vi "Att configurações.vi"(0 "Entrada de Configurações":T1={"Simulações"={"Nível Qualidade"="Ótima", "Turno"="Turno 1"}, "Captura de Imagens"={"Pasta com imagens"=path "", "Mostrar imagens capturadas"=FALSE}, "Caminhos"={"Arquivo de log"=path ""}}, 1 "Message Queue":refnum<queue>, 2 "Ler/Gravar":enum16{"Ler", "Gravar"}(ring), 3 "error in (no error)":errorcluster) -> (7 "Saída de configurações":T1={"Simulações"={"Nível Qualidade"="Ótima", "Turno"="Turno 1"}, "Captura de Imagens"={"Pasta com imagens"=path "", "Mostrar imagens capturadas"=FALSE}, "Caminhos"={"Arquivo de log"=path ""}}, 10 "error out":errorcluster)   [LabVIEW 2020, in "Configurações.lvlib"]
doc: "Executa ações definidas para cada configuração que existe no Type Def \"Configurações\".\n\nEsse VI não salva efetivamente as configurações no arquivo .ini ou na memória, ele somente adiciona na fila ações para cada configuração."
uses:
  Message Queue/Message Cluster.ctl
  <vilib>/Utility/config.llb/Read Key (String).vi
  <vilib>/Utility/config.llb/Write Key (String).vi
  Message Queue/Enqueue Message (Single).vi
  <vilib>/Utility/config.llb/Read Key (Boolean).vi
  <vilib>/Utility/config.llb/Read Key (Path).vi
  Message Queue/Message Queue.lvlib
  <vilib>/Utility/config.llb/NI_LVConfig.lvlib
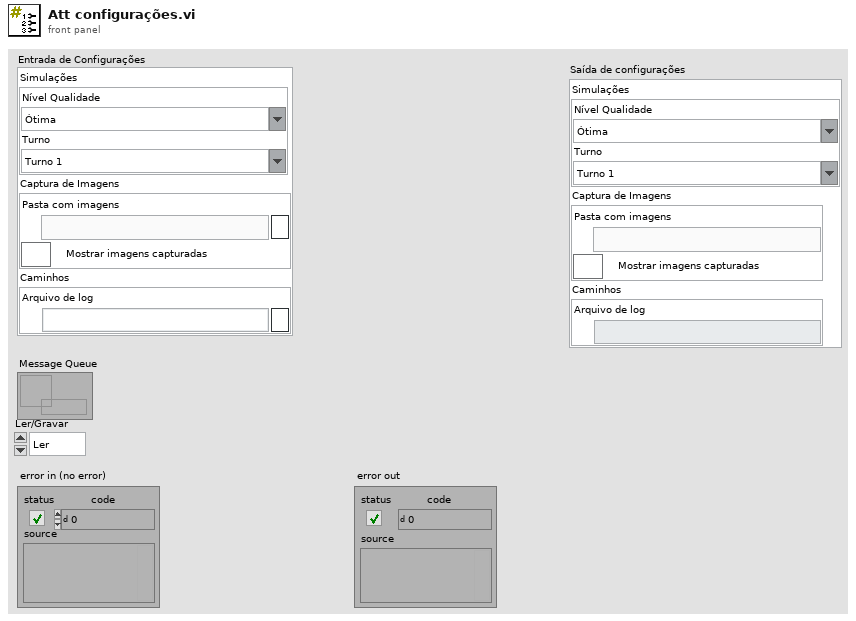
[diagram p1: front panel]
types:
  T1 = typedef "Configurações.lvlib/Configurações padrões.ctl" = cluster{"Simulações":cluster{"Nível Qualidade":string, "Turno":string}, "Captura de Imagens":cluster{"Pasta com imagens":path, "Mostrar imagens capturadas":bool}, "Caminhos":cluster{"Arquivo de log":path}}
  T2 = typedef "NI_LVConfig.lvlib/Config Data RefNum.ctl" = refnum<k1>
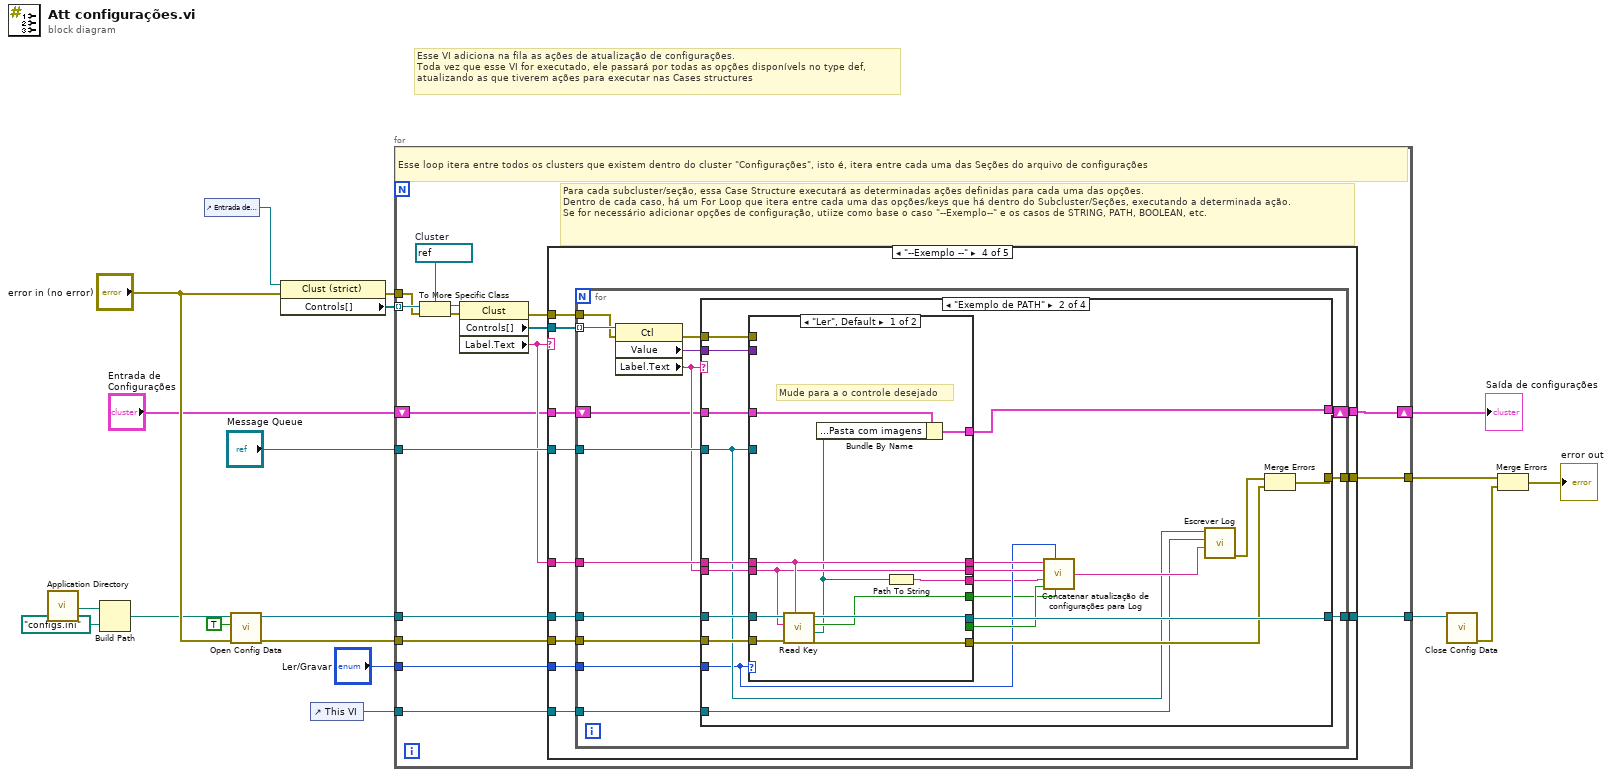
[diagram p0: block diagram]
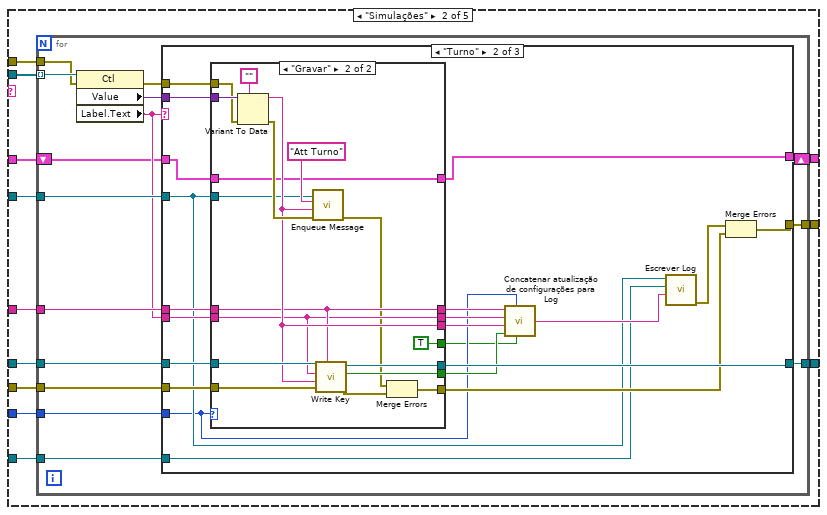
[diagram p3: hidden frame]
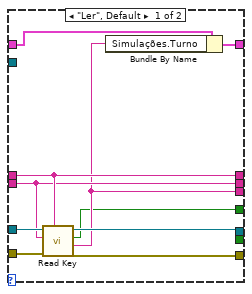
[diagram p5: hidden frame]
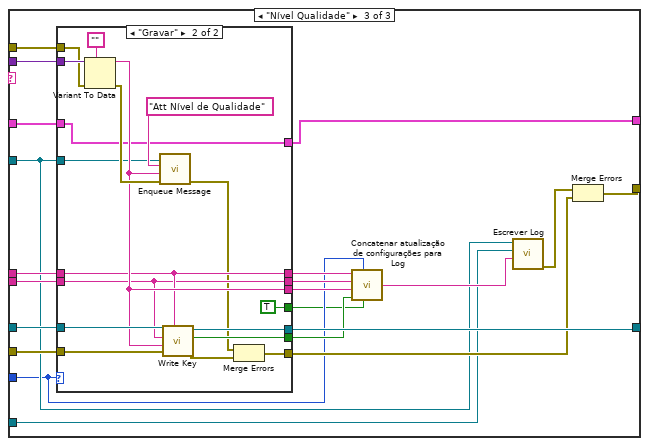
[diagram p6: hidden frame]
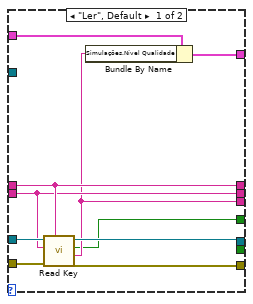
[diagram p7: hidden frame]
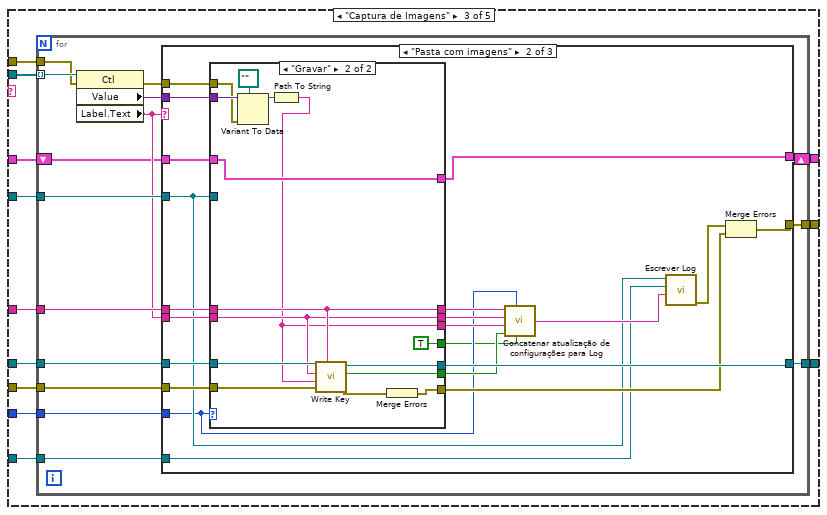
[diagram p8: hidden frame]
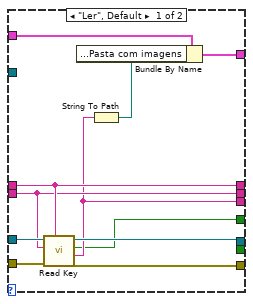
[diagram p10: hidden frame]
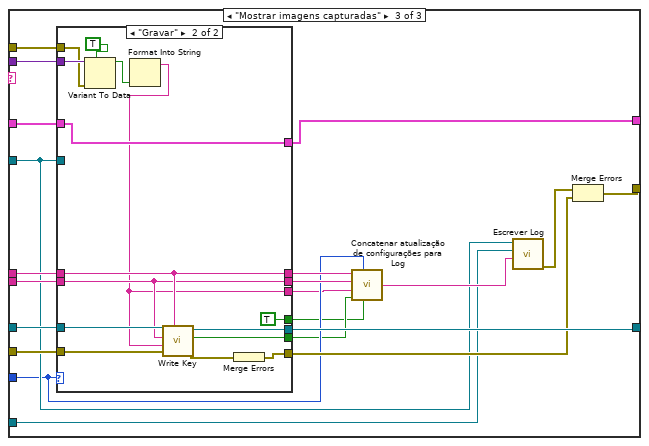
[diagram p11: hidden frame]
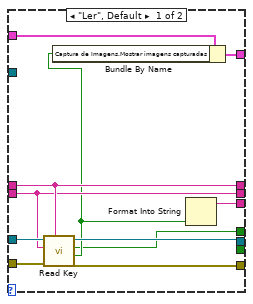
[diagram p12: hidden frame]
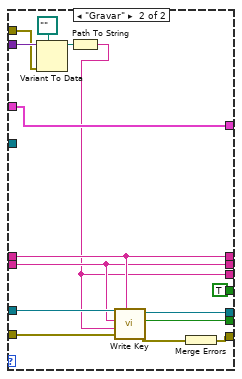
[diagram p14: hidden frame]
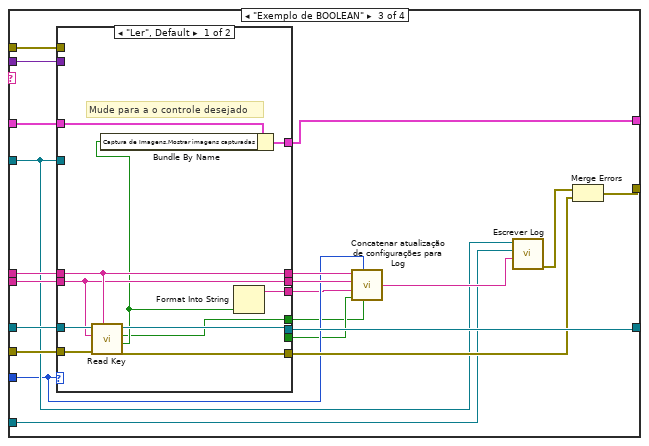
[diagram p15: hidden frame]
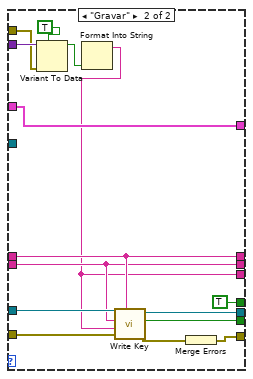
[diagram p16: hidden frame]
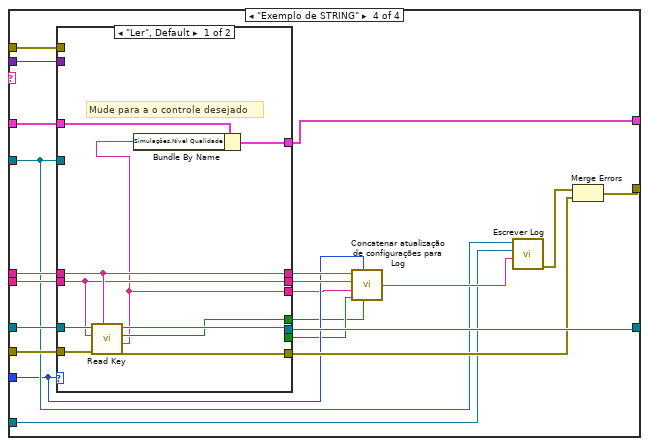
[diagram p17: hidden frame]
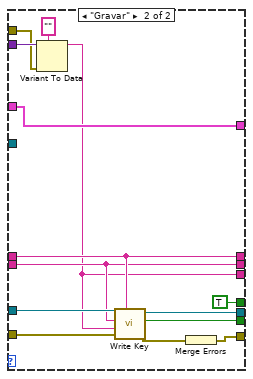
[diagram p18: hidden frame]
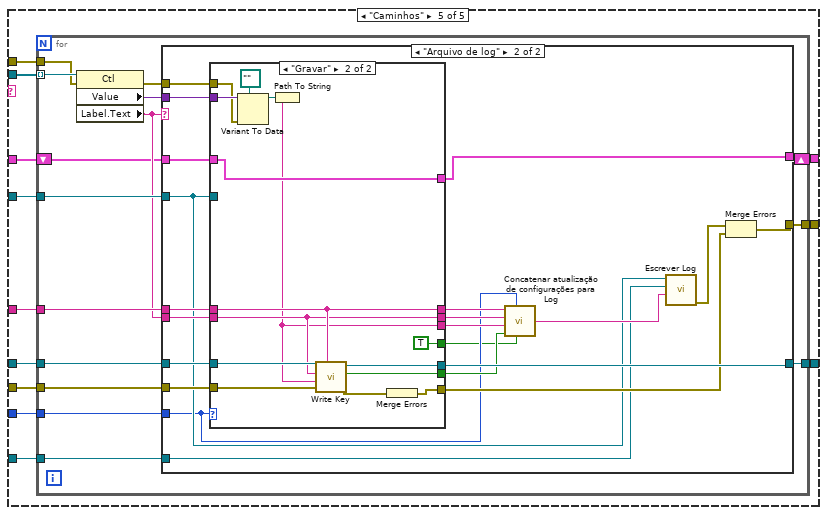
[diagram p19: hidden frame]
diagram:
  # "Esse VI adiciona na fila as ações de atualização de configurações.\nToda vez que esse VI for executado, ele passará por todas as opções disponívels no type def,\natualizando as que tiverem ações para executar nas Cases structures"
  n1 = call <vilib>:"Application Directory.vi"() -> ("Application Directory"=w2:path)
  n2 = Build Path(base path=w2, name or relative path=path "configs.ini") -> (appended path=w1:path)
  n3 = control-ref of="Entrada de Configurações"() -> (w16:refnum<vi>)
  n4 = call <vilib>:"Open Config Data.vi"("error in (no error)"="error in (no error)", "create file if necessary (T)"=TRUE, "configuration file path"=w1) -> ("error out"=w11:errorcluster, "refnum"=w13:T2)  [unwired: 6 in, 1 out]
  n5 = property on="Property Node" class="Clust (strict)"(reference=w16, error in="error in (no error)") -> (error out=w19:errorcluster, "Controls[]"=w18:refnum<vi>[])  [unwired: 1 out]
  n6 = control-ref of="This VI"() -> (w7:refnum<vi>)
  n7 = for {
    tunnel: w18 -> [w36] mode=indexing
    tunnel: w19 -> [w35]
    tunnel: "Message Queue" -> [w29]
    tunnel: [w28] -> w10
    tunnel: w13 -> [w27]
    tunnel: [w26] -> w12
    tunnel: w11 -> [w25]
    tunnel: w7 -> [w23]
    tunnel: "Ler/Gravar" -> [w22]
    shift-right: [w20] -> w4
    shift-left: "Entrada de Configurações" -> [w21]
    w34 = refnum<vi> refnum  # Cluster
    # "Para cada subcluster/seção, essa Case Structure executará as determinadas ações definidas para cada uma das opções.\nDentro de cada caso, há um For Loop que itera entre cada uma das opções/keys que há dentro do Subcluster/Seções, executando a determinada ação.\nSe for necessário adicionar opções de configuração, utiize como base o caso \"--Exemplo--\" e os casos de STRING, PATH, BOOLEAN, etc."
    # "Esse loop itera entre todos os clusters que existem dentro do cluster \"Configurações\", isto é, itera entre cada uma das Seções do arquivo de configurações"
    n8 = To More Specific Class(target class=w34, reference=w36, error in=w35) -> (specific class reference=w33:refnum<vi>, error out=w32:errorcluster)
    n9 = property class="Clust"(reference=w33, error in=w32) -> (error out=w30:errorcluster, "Controls[]"=w31:refnum<vi>[], "Label.Text"=w24:string)  [unwired: 1 out]
    n10 = case shown="\"--Exemplo --\"" w24 {
      tunnel: w31 -> [_ w51 w179 w303 w472]
      tunnel: w30 -> [w39 w50 w178 w302 w471]
      tunnel: w29 -> [_ w49 w177 w301 w470]
      tunnel: [w39 w48 w176 w300 w469] -> w28
      tunnel: w27 -> [w38 w47 w175 w299 w468]
      tunnel: [w38 w46 w174 w298 w467] -> w26
      tunnel: w25 -> [_ w45 w173 w297 w466]
      tunnel: w24 -> [_ w44 w172 w296 w465]
      tunnel: w23 -> [_ w43 w171 w295 w464]
      tunnel: w22 -> [_ w42 w170 w294 w463]
      tunnel: w21 -> [w37 w41 w169 w293 w462]
      tunnel: [w37 w40 w168 w292 w461] -> w20
      frame "Qualquer outra opção", Default {
      }
      frame "Simulações" {
        n11 = for {
          tunnel: w51 -> [w66] mode=indexing
          tunnel: w50 -> [w65]
          tunnel: w49 -> [w64]
          tunnel: [w61] -> w48
          tunnel: w47 -> [w60]
          tunnel: [w59] -> w46
          tunnel: w45 -> [w58]
          tunnel: w44 -> [w57]
          tunnel: w43 -> [w55]
          tunnel: w42 -> [w54]
          shift-right: [w52] -> w40
          shift-left: w41 -> [w53]
          n12 = property class="Ctl"(reference=w66, error in=w65) -> (error out=w62:errorcluster, "Value"=w63:variant, "Label.Text"=w56:string)  [unwired: 1 out]
          n13 = case shown="\"Turno\"" w56 {
            tunnel: w64 -> [_ w75 w124]
            tunnel: w63 -> [_ w90 w139]
            tunnel: w62 -> [w69 w89 w138]
            tunnel: [w69 w80 w129] -> w61
            tunnel: w60 -> [w68 w88 w137]
            tunnel: [w68 w87 w136] -> w59
            tunnel: w58 -> [_ w86 w135]
            tunnel: w57 -> [_ w83 w132]
            tunnel: w56 -> [_ w82 w131]
            tunnel: w55 -> [_ w74 w123]
            tunnel: w54 -> [_ w73 w122]
            tunnel: w53 -> [w67 w72 w121]
            tunnel: [w67 w71 w120] -> w52
            frame "Qualquer outra opção", Default {
            }
            frame "Turno" {
              n14 = case shown="\"Gravar\"" w73 {
                tunnel: w90 -> [_ w118]
                tunnel: w89 -> [_ w116]
                tunnel: w88 -> [w100 w113]
                tunnel: [w99 w112] -> w87
                tunnel: w86 -> [w97 w111]
                tunnel: [_ w110] -> w84
                tunnel: w83 -> [w96 w107]
                tunnel: w82 -> [w95 w106]
                tunnel: [w93 w109] -> w81
                tunnel: [w98 w104] -> w78
                tunnel: w75 -> [_ w108]
                tunnel: [w96 w107] -> w77
                tunnel: [w95 w106] -> w76
                tunnel: [w94 w102] -> w71
                tunnel: w72 -> [w92 w102]
                tunnel: [w91 TRUE ("found?")] -> w70
                frame "Ler", Default {
                  n15 = call-poly <vilib>:"Read Key.vi"("section"=w96, "error in (no error)"=w97, "key"=w95, "refnum"=w100) -> ("error out"=w98:errorcluster, "value"=w93:string, "found?"=w91:bool, "refnum out"=w99:T2)  [unwired: 4 in]
                  n16 = Bundle By Name(cluster=w92, "Simulações.Turno"=w93) -> (w94:T1)
                }
                frame "Gravar" {
                  n17 = Variant To Data(error in=w116, type="", Variant=w118) -> (data=w109:string, error out=w115:errorcluster)
                  n18 = call-poly "Enqueue Message.vi"("error in (no error)"=w115, "Message Data"=w109, "Message"="Att Turno", "Message Queue"=w108) -> ("error out"=w103:errorcluster)  [unwired: 6 in, 1 out]
                  n19 = call-poly <vilib>:"Write Key.vi"("section"=w107, "error in (no error)"=w111, "value"=w109, "key"=w106, "refnum"=w113) -> ("error out"=w105:errorcluster, "found?"=w110:bool, "refnum out"=w112:T2)  [unwired: 4 in]
                  n20 = Merge Errors(w103, w105) -> (w104:errorcluster)
                }
              }
              n21 = call "Concatenar atualização de configurações para Log.vi"("Seção/Key encontrada"=w70, "Leitura/Escrita"=w73, "Key ja existia?"=w84, "Valor"=w81, "Nome da Chave"=w76, "Nome da Seção"=w77) -> ("Texto Concatenado"=w85:string)
              n22 = call "Escrever Log.vi"("Dados para Log"=w85, "VI"=w74, "Queue in"=w75) -> ("error out"=w79:errorcluster)  [unwired: 7 in, 1 out]
              n23 = Merge Errors(w79, w78) -> (w80:errorcluster)
            }
            frame "Nível Qualidade" {
              n24 = case shown="\"Gravar\"" w122 {
                tunnel: w139 -> [_ w167]
                tunnel: w138 -> [_ w165]
                tunnel: w137 -> [w149 w162]
                tunnel: [w148 w161] -> w136
                tunnel: w135 -> [w146 w160]
                tunnel: [_ w159] -> w133
                tunnel: w132 -> [w145 w156]
                tunnel: w131 -> [w144 w155]
                tunnel: [w142 w158] -> w130
                tunnel: [w147 w153] -> w127
                tunnel: w124 -> [_ w157]
                tunnel: [w145 w156] -> w126
                tunnel: [w144 w155] -> w125
                tunnel: [w143 w151] -> w120
                tunnel: w121 -> [w141 w151]
                tunnel: [w140 TRUE ("found?")] -> w119
                frame "Ler", Default {
                  n25 = call-poly <vilib>:"Read Key.vi"("section"=w145, "error in (no error)"=w146, "key"=w144, "refnum"=w149) -> ("error out"=w147:errorcluster, "value"=w142:string, "found?"=w140:bool, "refnum out"=w148:T2)  [unwired: 4 in]
                  n26 = Bundle By Name(cluster=w141, "Simulações.Nível Qualidade"=w142) -> (w143:T1)
                }
                frame "Gravar" {
                  n27 = Variant To Data(error in=w165, type="", Variant=w167) -> (data=w158:string, error out=w164:errorcluster)
                  n28 = call-poly "Enqueue Message.vi"("error in (no error)"=w164, "Message Data"=w158, "Message"="Att Nível de Qualidade", "Message Queue"=w157) -> ("error out"=w152:errorcluster)  [unwired: 6 in, 1 out]
                  n29 = call-poly <vilib>:"Write Key.vi"("section"=w156, "error in (no error)"=w160, "value"=w158, "key"=w155, "refnum"=w162) -> ("error out"=w154:errorcluster, "found?"=w159:bool, "refnum out"=w161:T2)  [unwired: 4 in]
                  n30 = Merge Errors(w152, w154) -> (w153:errorcluster)
                }
              }
              n31 = call "Concatenar atualização de configurações para Log.vi"("Seção/Key encontrada"=w119, "Leitura/Escrita"=w122, "Key ja existia?"=w133, "Valor"=w130, "Nome da Chave"=w125, "Nome da Seção"=w126) -> ("Texto Concatenado"=w134:string)
              n32 = call "Escrever Log.vi"("Dados para Log"=w134, "VI"=w123, "Queue in"=w124) -> ("error out"=w128:errorcluster)  [unwired: 7 in, 1 out]
              n33 = Merge Errors(w128, w127) -> (w129:errorcluster)
            }
          }
        }
      }
      frame "Captura de Imagens" {
        n34 = for {
          tunnel: w179 -> [w194] mode=indexing
          tunnel: w178 -> [w193]
          tunnel: w177 -> [w192]
          tunnel: [w189] -> w176
          tunnel: w175 -> [w188]
          tunnel: [w187] -> w174
          tunnel: w173 -> [w186]
          tunnel: w172 -> [w185]
          tunnel: w171 -> [w183]
          tunnel: w170 -> [w182]
          shift-right: [w180] -> w168
          shift-left: w169 -> [w181]
          n35 = property class="Ctl"(reference=w194, error in=w193) -> (error out=w190:errorcluster, "Value"=w191:variant, "Label.Text"=w184:string)  [unwired: 1 out]
          n36 = case shown="\"Pasta com imagens\"" w184 {
            tunnel: w192 -> [_ w203 w252]
            tunnel: w191 -> [_ w218 w265]
            tunnel: w190 -> [w197 w217 w264]
            tunnel: [w197 w208 w257] -> w189
            tunnel: w188 -> [w196 w216 w263]
            tunnel: [w196 w215 w262] -> w187
            tunnel: w186 -> [_ w214 w261]
            tunnel: w185 -> [_ w211 w259]
            tunnel: w184 -> [_ w210 w258]
            tunnel: w183 -> [_ w202 w251]
            tunnel: w182 -> [_ w201 w250]
            tunnel: w181 -> [w195 w200 w249]
            tunnel: [w195 w199 w248] -> w180
            frame "Qualquer outra opção", Default {
            }
            frame "Pasta com imagens" {
              n37 = case shown="\"Gravar\"" w201 {
                tunnel: w218 -> [_ w244]
                tunnel: w217 -> [_ w243]
                tunnel: w216 -> [w229 w242]
                tunnel: [w228 w241] -> w215
                tunnel: w214 -> [w226 w240]
                tunnel: [_ w239] -> w212
                tunnel: w211 -> [w225 w238]
                tunnel: w210 -> [w224 w237]
                tunnel: [w220 w230] -> w209
                tunnel: [w227 w235] -> w206
                tunnel: w203 -> [_ _]
                tunnel: [w225 w238] -> w205
                tunnel: [w224 w237] -> w204
                tunnel: [w223 w234] -> w199
                tunnel: w200 -> [w222 w234]
                tunnel: [w219 TRUE ("found?")] -> w198
                frame "Ler", Default {
                  n38 = call-poly <vilib>:"Read Key.vi"("section"=w225, "error in (no error)"=w226, "key"=w224, "refnum"=w229) -> ("error out"=w227:errorcluster, "value"=w220:string, "found?"=w219:bool, "refnum out"=w228:T2)  [unwired: 4 in]
                  n39 = String To Path(string=w220) -> (path=w221:path)
                  n40 = Bundle By Name(cluster=w222, "Captura de Imagens.Pasta com imagens"=w221) -> (w223:T1)
                }
                frame "Gravar" {
                  n41 = Variant To Data(error in=w243, type=path "", Variant=w244) -> (data=w231:path)  [unwired: 1 out]
                  n42 = Path To String(path=w231) -> (string=w230:string)
                  n43 = call-poly <vilib>:"Write Key.vi"("section"=w238, "error in (no error)"=w240, "value"=w230, "key"=w237, "refnum"=w242) -> ("error out"=w236:errorcluster, "found?"=w239:bool, "refnum out"=w241:T2)  [unwired: 4 in]
                  n44 = Merge Errors(w236) -> (w235:errorcluster)
                }
              }
              n45 = call "Concatenar atualização de configurações para Log.vi"("Seção/Key encontrada"=w198, "Leitura/Escrita"=w201, "Key ja existia?"=w212, "Valor"=w209, "Nome da Chave"=w204, "Nome da Seção"=w205) -> ("Texto Concatenado"=w213:string)
              n46 = call "Escrever Log.vi"("Dados para Log"=w213, "VI"=w202, "Queue in"=w203) -> ("error out"=w207:errorcluster)  [unwired: 7 in, 1 out]
              n47 = Merge Errors(w207, w206) -> (w208:errorcluster)
            }
            frame "Mostrar imagens capturadas" {
              n48 = case shown="\"Gravar\"" w250 {
                tunnel: w265 -> [_ w291]
                tunnel: w264 -> [_ w290]
                tunnel: w263 -> [w276 w289]
                tunnel: [w275 w288] -> w262
                tunnel: w261 -> [w273 w287]
                tunnel: [_ w286] -> w247
                tunnel: w259 -> [w272 w285]
                tunnel: w258 -> [w271 w284]
                tunnel: [w274 w282] -> w255
                tunnel: w252 -> [_ _]
                tunnel: [w272 w285] -> w254
                tunnel: [w271 w284] -> w253
                tunnel: [w270 w281] -> w248
                tunnel: w249 -> [w268 w281]
                tunnel: [w267 w277] -> w246
                tunnel: [w266 TRUE ("found?")] -> w245
                frame "Ler", Default {
                  n49 = call-poly <vilib>:"Read Key.vi"("section"=w272, "error in (no error)"=w273, "key"=w271, "refnum"=w276) -> ("error out"=w274:errorcluster, "value"=w269:bool, "found?"=w266:bool, "refnum out"=w275:T2)  [unwired: 4 in]
                  n50 = Bundle By Name(cluster=w268, "Captura de Imagens.Mostrar imagens capturadas"=w269) -> (w270:T1)
                  n51 = Format Into String(w269) -> (resulting string=w267:string)  [unwired: 3 in, 1 out]
                }
                frame "Gravar" {
                  n52 = Variant To Data(error in=w290, type=TRUE, Variant=w291) -> (data=w278:bool)  [unwired: 1 out]
                  n53 = Format Into String(w278) -> (resulting string=w277:string)  [unwired: 3 in, 1 out]
                  n54 = call-poly <vilib>:"Write Key.vi"("section"=w285, "error in (no error)"=w287, "value"=w277, "key"=w284, "refnum"=w289) -> ("error out"=w283:errorcluster, "found?"=w286:bool, "refnum out"=w288:T2)  [unwired: 4 in]
                  n55 = Merge Errors(w283) -> (w282:errorcluster)
                }
              }
              n56 = call "Concatenar atualização de configurações para Log.vi"("Seção/Key encontrada"=w245, "Leitura/Escrita"=w250, "Key ja existia?"=w247, "Valor"=w246, "Nome da Chave"=w253, "Nome da Seção"=w254) -> ("Texto Concatenado"=w260:string)
              n57 = call "Escrever Log.vi"("Dados para Log"=w260, "VI"=w251, "Queue in"=w252) -> ("error out"=w256:errorcluster)  [unwired: 7 in, 1 out]
              n58 = Merge Errors(w256, w255) -> (w257:errorcluster)
            }
          }
        }
      }
      frame "--Exemplo --" {
        n59 = for {
          tunnel: w303 -> [w318] mode=indexing
          tunnel: w302 -> [w317]
          tunnel: w301 -> [w316]
          tunnel: [w313] -> w300
          tunnel: w299 -> [w312]
          tunnel: [w311] -> w298
          tunnel: w297 -> [w310]
          tunnel: w296 -> [w309]
          tunnel: w295 -> [w307]
          tunnel: w294 -> [w306]
          shift-right: [w304] -> w292
          shift-left: w293 -> [w305]
          n60 = property class="Ctl"(reference=w318, error in=w317) -> (error out=w314:errorcluster, "Value"=w315:variant, "Label.Text"=w308:string)  [unwired: 1 out]
          n61 = case shown="\"Exemplo de PATH\"" w308 {
            tunnel: w316 -> [_ w328 w376 w423]
            tunnel: w315 -> [_ w342 w389 w436]
            tunnel: w314 -> [w321 w341 w388 w435]
            tunnel: [w321 w333 w381 w428] -> w313
            tunnel: w312 -> [w320 w340 w387 w434]
            tunnel: [w320 w339 w386 w433] -> w311
            tunnel: w310 -> [_ w338 w385 w432]
            tunnel: w309 -> [_ w335 w383 w430]
            tunnel: w308 -> [_ w334 w382 w429]
            tunnel: w307 -> [_ w327 w375 w422]
            tunnel: w306 -> [_ w326 w374 w421]
            tunnel: w305 -> [w319 w325 w373 w420]
            tunnel: [w319 w324 w372 w419] -> w304
            frame "Qualquer outra opção", Default {
            }
            frame "Exemplo de PATH" {
              n62 = case shown="\"Ler\", Default" w326 {
                tunnel: w342 -> [_ w368]
                tunnel: w341 -> [_ w367]
                tunnel: w340 -> [w353 w366]
                tunnel: [w352 w365] -> w339
                tunnel: w338 -> [w350 w364]
                tunnel: [_ w363] -> w336
                tunnel: w335 -> [w349 w362]
                tunnel: w334 -> [w348 w361]
                tunnel: [w351 w359] -> w331
                tunnel: w328 -> [_ _]
                tunnel: [w349 w362] -> w330
                tunnel: [w348 w361] -> w329
                tunnel: [w347 w358] -> w324
                tunnel: w325 -> [w346 w358]
                tunnel: [w345 TRUE ("found?")] -> w323
                tunnel: [w343 w354] -> w322
                frame "Ler", Default {
                  # "Mude para a o controle desejado"
                  n63 = call-poly <vilib>:"Read Key.vi"("section"=w349, "error in (no error)"=w350, "key"=w348, "refnum"=w353) -> ("error out"=w351:errorcluster, "value"=w344:path, "found?"=w345:bool, "refnum out"=w352:T2)  [unwired: 4 in]
                  n64 = Bundle By Name(cluster=w346, "Captura de Imagens.Pasta com imagens"=w344) -> (w347:T1)
                  n65 = Path To String(path=w344) -> (string=w343:string)
                }
                frame "Gravar" {
                  n66 = Variant To Data(error in=w367, type=path "", Variant=w368) -> (data=w355:path)  [unwired: 1 out]
                  n67 = Path To String(path=w355) -> (string=w354:string)
                  n68 = call-poly <vilib>:"Write Key.vi"("section"=w362, "error in (no error)"=w364, "value"=w354, "key"=w361, "refnum"=w366) -> ("error out"=w360:errorcluster, "found?"=w363:bool, "refnum out"=w365:T2)  [unwired: 4 in]
                  n69 = Merge Errors(w360) -> (w359:errorcluster)
                }
              }
              n70 = call "Concatenar atualização de configurações para Log.vi"("Seção/Key encontrada"=w323, "Leitura/Escrita"=w326, "Key ja existia?"=w336, "Valor"=w322, "Nome da Chave"=w329, "Nome da Seção"=w330) -> ("Texto Concatenado"=w337:string)
              n71 = call "Escrever Log.vi"("Dados para Log"=w337, "VI"=w327, "Queue in"=w328) -> ("error out"=w332:errorcluster)  [unwired: 7 in, 1 out]
              n72 = Merge Errors(w332, w331) -> (w333:errorcluster)
            }
            frame "Exemplo de BOOLEAN" {
              n73 = case shown="\"Ler\", Default" w374 {
                tunnel: w389 -> [_ w415]
                tunnel: w388 -> [_ w414]
                tunnel: w387 -> [w400 w413]
                tunnel: [w399 w412] -> w386
                tunnel: w385 -> [w397 w411]
                tunnel: [_ w410] -> w371
                tunnel: w383 -> [w396 w409]
                tunnel: w382 -> [w395 w408]
                tunnel: [w398 w406] -> w379
                tunnel: w376 -> [_ _]
                tunnel: [w396 w409] -> w378
                tunnel: [w395 w408] -> w377
                tunnel: [w394 w405] -> w372
                tunnel: w373 -> [w392 w405]
                tunnel: [w391 w401] -> w370
                tunnel: [w390 TRUE ("found?")] -> w369
                frame "Ler", Default {
                  # "Mude para a o controle desejado"
                  n74 = call-poly <vilib>:"Read Key.vi"("section"=w396, "error in (no error)"=w397, "key"=w395, "refnum"=w400) -> ("error out"=w398:errorcluster, "value"=w393:bool, "found?"=w390:bool, "refnum out"=w399:T2)  [unwired: 4 in]
                  n75 = Bundle By Name(cluster=w392, "Captura de Imagens.Mostrar imagens capturadas"=w393) -> (w394:T1)
                  n76 = Format Into String(w393) -> (resulting string=w391:string)  [unwired: 3 in, 1 out]
                }
                frame "Gravar" {
                  n77 = Variant To Data(error in=w414, type=TRUE, Variant=w415) -> (data=w402:bool)  [unwired: 1 out]
                  n78 = Format Into String(w402) -> (resulting string=w401:string)  [unwired: 3 in, 1 out]
                  n79 = call-poly <vilib>:"Write Key.vi"("section"=w409, "error in (no error)"=w411, "value"=w401, "key"=w408, "refnum"=w413) -> ("error out"=w407:errorcluster, "found?"=w410:bool, "refnum out"=w412:T2)  [unwired: 4 in]
                  n80 = Merge Errors(w407) -> (w406:errorcluster)
                }
              }
              n81 = call "Concatenar atualização de configurações para Log.vi"("Seção/Key encontrada"=w369, "Leitura/Escrita"=w374, "Key ja existia?"=w371, "Valor"=w370, "Nome da Chave"=w377, "Nome da Seção"=w378) -> ("Texto Concatenado"=w384:string)
              n82 = call "Escrever Log.vi"("Dados para Log"=w384, "VI"=w375, "Queue in"=w376) -> ("error out"=w380:errorcluster)  [unwired: 7 in, 1 out]
              n83 = Merge Errors(w380, w379) -> (w381:errorcluster)
            }
            frame "Exemplo de STRING" {
              n84 = case shown="\"Ler\", Default" w421 {
                tunnel: w436 -> [_ w460]
                tunnel: w435 -> [_ w459]
                tunnel: w434 -> [w446 w458]
                tunnel: [w445 w457] -> w433
                tunnel: w432 -> [w443 w456]
                tunnel: [_ w455] -> w418
                tunnel: w430 -> [w442 w454]
                tunnel: w429 -> [w441 w453]
                tunnel: [w444 w451] -> w426
                tunnel: w423 -> [_ _]
                tunnel: [w442 w454] -> w425
                tunnel: [w441 w453] -> w424
                tunnel: [w440 w450] -> w419
                tunnel: w420 -> [w439 w450]
                tunnel: [w437 w447] -> w417
                tunnel: [w438 TRUE ("found?")] -> w416
                frame "Ler", Default {
                  # "Mude para a o controle desejado"
                  n85 = call-poly <vilib>:"Read Key.vi"("section"=w442, "error in (no error)"=w443, "key"=w441, "refnum"=w446) -> ("error out"=w444:errorcluster, "value"=w437:string, "found?"=w438:bool, "refnum out"=w445:T2)  [unwired: 4 in]
                  n86 = Bundle By Name(cluster=w439, "Simulações.Nível Qualidade"=w437) -> (w440:T1)
                }
                frame "Gravar" {
                  n87 = Variant To Data(error in=w459, type="", Variant=w460) -> (data=w447:string)  [unwired: 1 out]
                  n88 = call-poly <vilib>:"Write Key.vi"("section"=w454, "error in (no error)"=w456, "value"=w447, "key"=w453, "refnum"=w458) -> ("error out"=w452:errorcluster, "found?"=w455:bool, "refnum out"=w457:T2)  [unwired: 4 in]
                  n89 = Merge Errors(w452) -> (w451:errorcluster)
                }
              }
              n90 = call "Concatenar atualização de configurações para Log.vi"("Seção/Key encontrada"=w416, "Leitura/Escrita"=w421, "Key ja existia?"=w418, "Valor"=w417, "Nome da Chave"=w424, "Nome da Seção"=w425) -> ("Texto Concatenado"=w431:string)
              n91 = call "Escrever Log.vi"("Dados para Log"=w431, "VI"=w422, "Queue in"=w423) -> ("error out"=w427:errorcluster)  [unwired: 7 in, 1 out]
              n92 = Merge Errors(w427, w426) -> (w428:errorcluster)
            }
          }
        }
      }
      frame "Caminhos" {
        n93 = for {
          tunnel: w472 -> [w487] mode=indexing
          tunnel: w471 -> [w486]
          tunnel: w470 -> [w485]
          tunnel: [w482] -> w469
          tunnel: w468 -> [w481]
          tunnel: [w480] -> w467
          tunnel: w466 -> [w479]
          tunnel: w465 -> [w478]
          tunnel: w464 -> [w476]
          tunnel: w463 -> [w475]
          shift-right: [w473] -> w461
          shift-left: w462 -> [w474]
          n94 = property class="Ctl"(reference=w487, error in=w486) -> (error out=w483:errorcluster, "Value"=w484:variant, "Label.Text"=w477:string)  [unwired: 1 out]
          n95 = case shown="\"Arquivo de log\"" w477 {
            tunnel: w485 -> [_ w496]
            tunnel: w484 -> [_ w511]
            tunnel: w483 -> [w490 w510]
            tunnel: [w490 w501] -> w482
            tunnel: w481 -> [w489 w509]
            tunnel: [w489 w508] -> w480
            tunnel: w479 -> [_ w507]
            tunnel: w478 -> [_ w504]
            tunnel: w477 -> [_ w503]
            tunnel: w476 -> [_ w495]
            tunnel: w475 -> [_ w494]
            tunnel: w474 -> [w488 w493]
            tunnel: [w488 w492] -> w473
            frame "Qualquer outra opção", Default {
            }
            frame "Arquivo de log" {
              n96 = case shown="\"Gravar\"" w494 {
                tunnel: w511 -> [_ w537]
                tunnel: w510 -> [_ w536]
                tunnel: w509 -> [w522 w535]
                tunnel: [w521 w534] -> w508
                tunnel: w507 -> [w519 w533]
                tunnel: [_ w532] -> w505
                tunnel: w504 -> [w518 w531]
                tunnel: w503 -> [w517 w530]
                tunnel: [w513 w523] -> w502
                tunnel: [w520 w528] -> w499
                tunnel: w496 -> [_ _]
                tunnel: [w518 w531] -> w498
                tunnel: [w517 w530] -> w497
                tunnel: [w516 w527] -> w492
                tunnel: w493 -> [w515 w527]
                tunnel: [w512 TRUE ("found?")] -> w491
                frame "Ler", Default {
                  n97 = call-poly <vilib>:"Read Key.vi"("section"=w518, "error in (no error)"=w519, "key"=w517, "refnum"=w522) -> ("error out"=w520:errorcluster, "value"=w513:string, "found?"=w512:bool, "refnum out"=w521:T2)  [unwired: 4 in]
                  n98 = String To Path(string=w513) -> (path=w514:path)
                  n99 = Bundle By Name(cluster=w515, "Caminhos.Arquivo de log"=w514) -> (w516:T1)
                }
                frame "Gravar" {
                  n100 = Variant To Data(error in=w536, type=path "", Variant=w537) -> (data=w524:path)  [unwired: 1 out]
                  n101 = Path To String(path=w524) -> (string=w523:string)
                  n102 = call-poly <vilib>:"Write Key.vi"("section"=w531, "error in (no error)"=w533, "value"=w523, "key"=w530, "refnum"=w535) -> ("error out"=w529:errorcluster, "found?"=w532:bool, "refnum out"=w534:T2)  [unwired: 4 in]
                  n103 = Merge Errors(w529) -> (w528:errorcluster)
                }
              }
              n104 = call "Concatenar atualização de configurações para Log.vi"("Seção/Key encontrada"=w491, "Leitura/Escrita"=w494, "Key ja existia?"=w505, "Valor"=w502, "Nome da Chave"=w497, "Nome da Seção"=w498) -> ("Texto Concatenado"=w506:string)
              n105 = call "Escrever Log.vi"("Dados para Log"=w506, "VI"=w495, "Queue in"=w496) -> ("error out"=w500:errorcluster)  [unwired: 7 in, 1 out]
              n106 = Merge Errors(w500, w499) -> (w501:errorcluster)
            }
          }
        }
      }
    }
  }
  "Saída de configurações" <- w4
  n107 = call <vilib>:"Close Config Data.vi"("refnum"=w12) -> ("error out"=w8:errorcluster)  [unwired: 9 in, 1 out]
  n108 = Merge Errors(w10, w8) -> (→"error out":errorcluster)
